vi "test16.vi"() -> ()   [LabVIEW 2018]
uses:
  <vilib>/Instr/_visa.llb/VISA Configure Serial Port (Instr).vi
panel:
  in  "发送波特率":u32=9600
  in  "接收波特率":u32=9600
  out "是否收到":bool
  in  "停止":bool
  in  "保存按钮":bool=TRUE
  out "时间":string="2019/12/25\t13:20:46"
  in  "VISA receive":refnum<visa-resource-name>="COM7" caption="VISAreceive"
  in  "接收数据":bool=TRUE
  out "读取缓冲区1":string
  in  "点击发送":bool
  in  "写入缓冲区":string
  in  "VISA send":refnum<visa-resource-name>="COM7" caption="VISAsend"
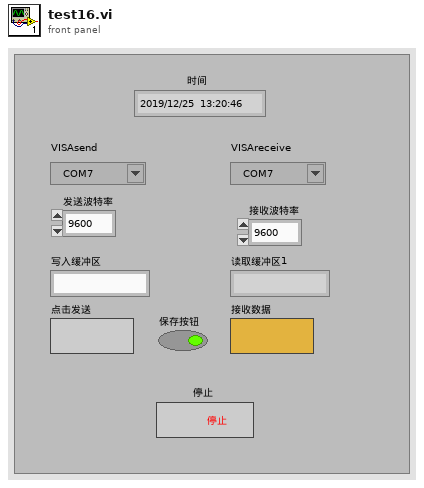
[diagram p1: front panel]
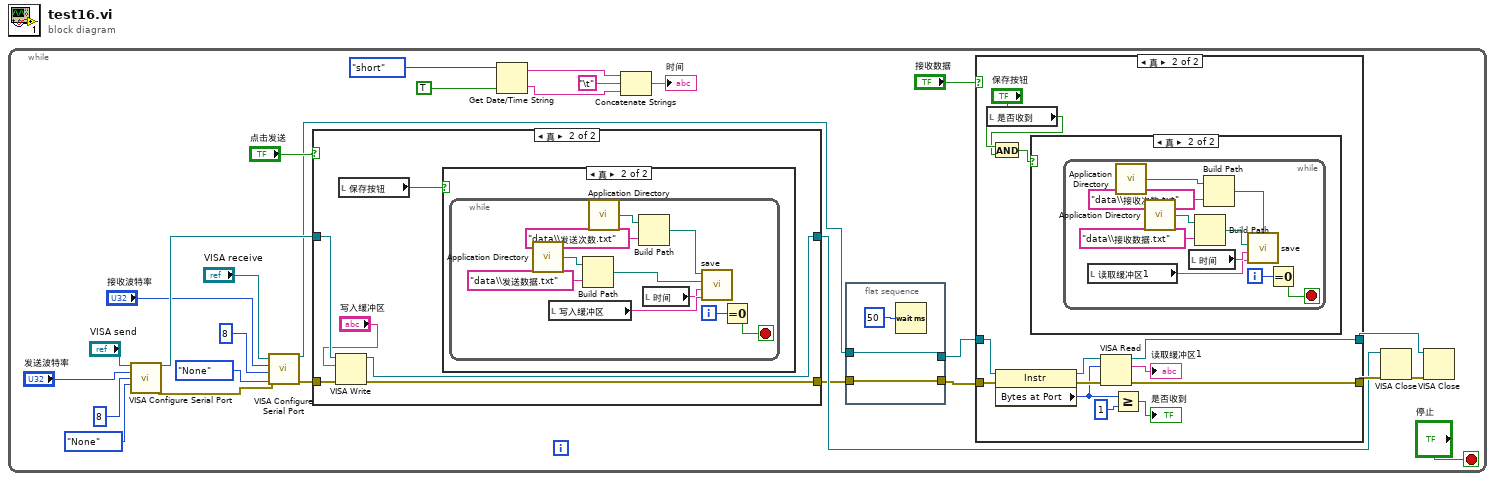
[diagram p0: block diagram]
diagram:
  n1 = while {
    stop <- "停止" stop-if-true
    n2 = call-poly "VISA Configure Serial Port"("VISA resource name"="VISA send", "baud rate (9600)"="发送波特率", "data bits (8)"=u16 8, "parity (0:none)"=enum16{"None", "Odd", "Even", "Mark", "Space"}."None") -> ("VISA resource name out"=w23:refnum<visa-resource-name>, "error out"=w9:errorcluster)  [unwired: 10 in]
    n3 = call-poly "VISA Configure Serial Port"("VISA resource name"="VISA receive", "baud rate (9600)"="接收波特率", "data bits (8)"=u16 8, "parity (0:none)"=enum16{"None", "Odd", "Even", "Mark", "Space"}."None", "error in (no error)"=w9) -> ("VISA resource name out"=w1:refnum<visa-resource-name>, "error out"=w8:errorcluster)  [unwired: 9 in]
    n4 = case shown="真" "点击发送" {
      tunnel: [w58 w64] -> w6
      tunnel: [w57 w61] -> w3
      tunnel: w23 -> [w58 w63]
      tunnel: w8 -> [w57 w60]
      frame False {
      }
      frame True {
        n5 = VISA Write(VISA resource name=w63, write buffer="写入缓冲区", error in (no error)=w60) -> (VISA resource name out=w64:refnum<visa-resource-name>, error out=w61:errorcluster)  [unwired: 1 out]
        n6 = local read "保存按钮"() -> (w62:bool)
        n7 = case shown="真" w62 {
          frame False {
          }
          frame True {
            n8 = while {
              i -> [w74]
              stop <- w73 stop-if-true
              n9 = call <vilib>:"Application Directory.vi"() -> ("Application Directory"=w67:path)
              n10 = local read "写入缓冲区"() -> (w72:string)
              n11 = Build Path(base path=w67, name or relative path="data\\发送数据.txt" ("名称或相对路径")) -> (appended path=w65:path)
              n12 = call <vilib>:"Application Directory.vi"() -> ("Application Directory"=w70:path)
              n13 = Build Path(base path=w70, name or relative path="data\\发送次数.txt" ("名称或相对路径")) -> (appended path=w68:path)
              n14 = local read "时间"() -> (w71:string)
              n15 = call "save.vi"("存盘数据"=w72, "时间"=w71, "数据（使用对话框）"=w65, "次数（使用对话框）"=w68) -> ()
              n16 = Equal To 0?(x=w74) -> (x = 0?=w73:bool)
            }
          }
        }
      }
    }
    n17 = Get Date/Time String(date format (0)=enum16{"short", "long", "abbreviated"}."short" ("日期格式(0)"), want seconds? (F)=TRUE ("需要秒？(F)")) -> (date string=w13:string, time string=w12:string)  [unwired: 1 in]
    n18 = Concatenate Strings(w13, "\t", w12) -> (→"时间":string)
    n19 = flat-sequence {
      tunnel: w1 -> [w31]
      tunnel: [w31] -> w4
      tunnel: w3 -> [w30]
      tunnel: [w30] -> w2
      frame #0 {
        n20 = Wait (ms)(milliseconds to wait=u32 50 ("等待时间（毫秒）")) -> ()  [unwired: 1 out]
      }
    }
    n21 = case shown="真" "接收数据" {
      tunnel: [w32 w43] -> w21
      tunnel: [w33 w42] -> w5
      tunnel: w4 -> [w33 w41]
      tunnel: w2 -> [w32 w40]
      frame False {
      }
      frame True {
        n22 = local read "是否收到"() -> (w35:bool)
        n23 = And(x="保存按钮", y=w35) -> (x .and. y?=w34:bool)
        n24 = property class="Instr"(reference=w41, error in=w40) -> (reference out=w46:refnum<visa-resource-name>, error out=w45:errorcluster, "Bytes at Port"=w39:u32)
        n25 = case shown="真" w34 {
          frame False {
          }
          frame True {
            n26 = while {
              i -> [w56]
              stop <- w55 stop-if-true
              n27 = local read "读取缓冲区1"() -> (w53:string)
              n28 = call <vilib>:"Application Directory.vi"() -> ("Application Directory"=w52:path)
              n29 = call <vilib>:"Application Directory.vi"() -> ("Application Directory"=w50:path)
              n30 = local read "时间"() -> (w54:string)
              n31 = Build Path(base path=w50, name or relative path="data\\接收数据.txt" ("名称或相对路径")) -> (appended path=w48:path)
              n32 = Build Path(base path=w52, name or relative path="data\\接收次数.txt" ("名称或相对路径")) -> (appended path=w47:path)
              n33 = call "save.vi"("存盘数据"=w53, "时间"=w54, "数据（使用对话框）"=w48, "次数（使用对话框）"=w47) -> ()
              n34 = Equal To 0?(x=w56) -> (x = 0?=w55:bool)
            }
          }
        }
        n35 = VISA Read(VISA resource name=w46, byte count=w39, error in (no error)=w45) -> (VISA resource name out=w42:refnum<visa-resource-name>, read buffer=→"读取缓冲区1":string, error out=w43:errorcluster)  [unwired: 1 out]
        n36 = Greater Or Equal?(x=w39, y=u32 1) -> (x >= y?=→"是否收到":bool)
      }
    }
    n37 = VISA Close(VISA resource name=w6, error in (no error)=w21) -> (error out=w7:errorcluster)
    n38 = VISA Close(VISA resource name=w5, error in (no error)=w7) -> ()  [unwired: 1 out]
  }
